vi "Output Error.vi"(1 "Output":dbl[](array[numeric]), 2 "Target Output":dbl[](array[numeric])) -> (0 "End Error":dbl[](array[numeric]))   [LabVIEW 2009]
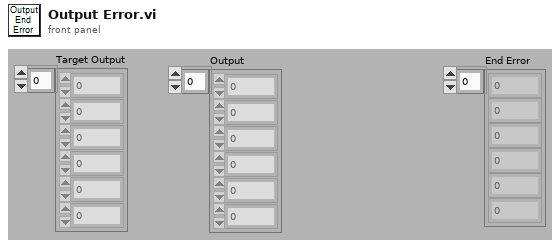
[diagram p1: front panel]
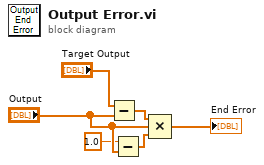
[diagram p0: block diagram]
diagram:
  n1 = Subtract(x="Target Output", y="Output") -> (x-y=w2:dbl[])
  n2 = Subtract(x=1.0, y="Output") -> (x-y=w5:dbl[])
  n3 = Compound Arithmetic op=MULTIPLY(w2, "Output", w5) -> (→"End Error":dbl[])
